vi "autonSample.vi"(0 "Auton Array":dbl[][](array[numeric]), 5 "LeftEncoder":dbl, 7 "RightEncoder":dbl, 11 "MeasuredHeading":dbl) -> (4 "Left Drive":dbl, 6 "Right Drive":dbl, 8 "Ramp ACT motor":dbl, 10 "Harvester":dbl, 13 "Shooter motor output":dbl, 14 "Turret Rotation":dbl, 15 "Convyeor":dbl)   [LabVIEW 2011]
uses:
  Robot Global Data.vi
panel:
  out "Primitive ID":i16
  out "Tzero":i64
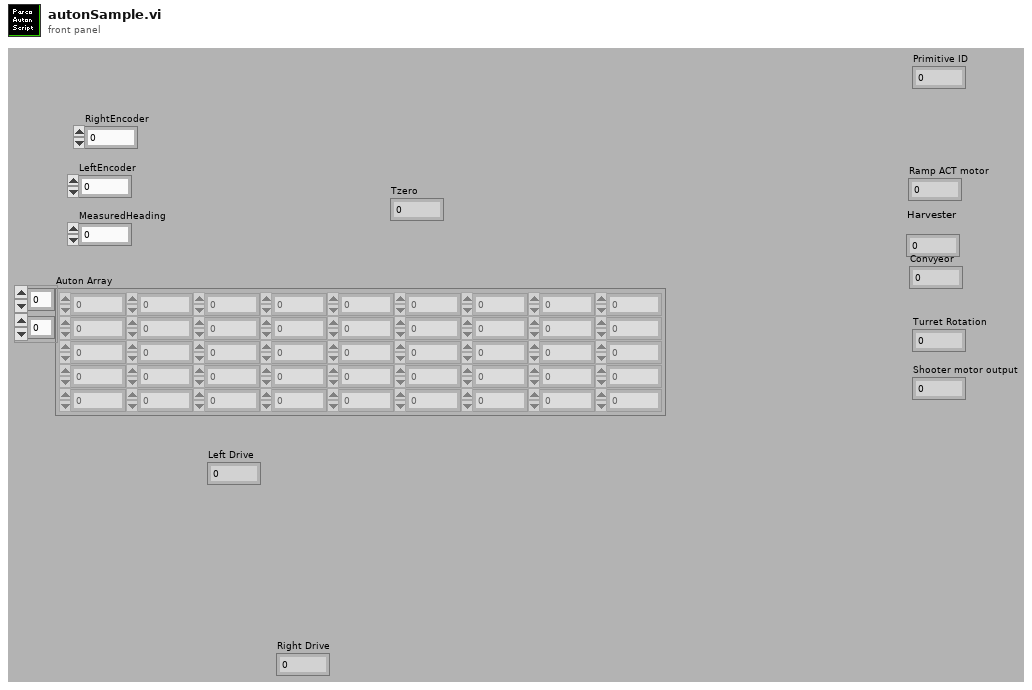
[diagram p1: front panel]
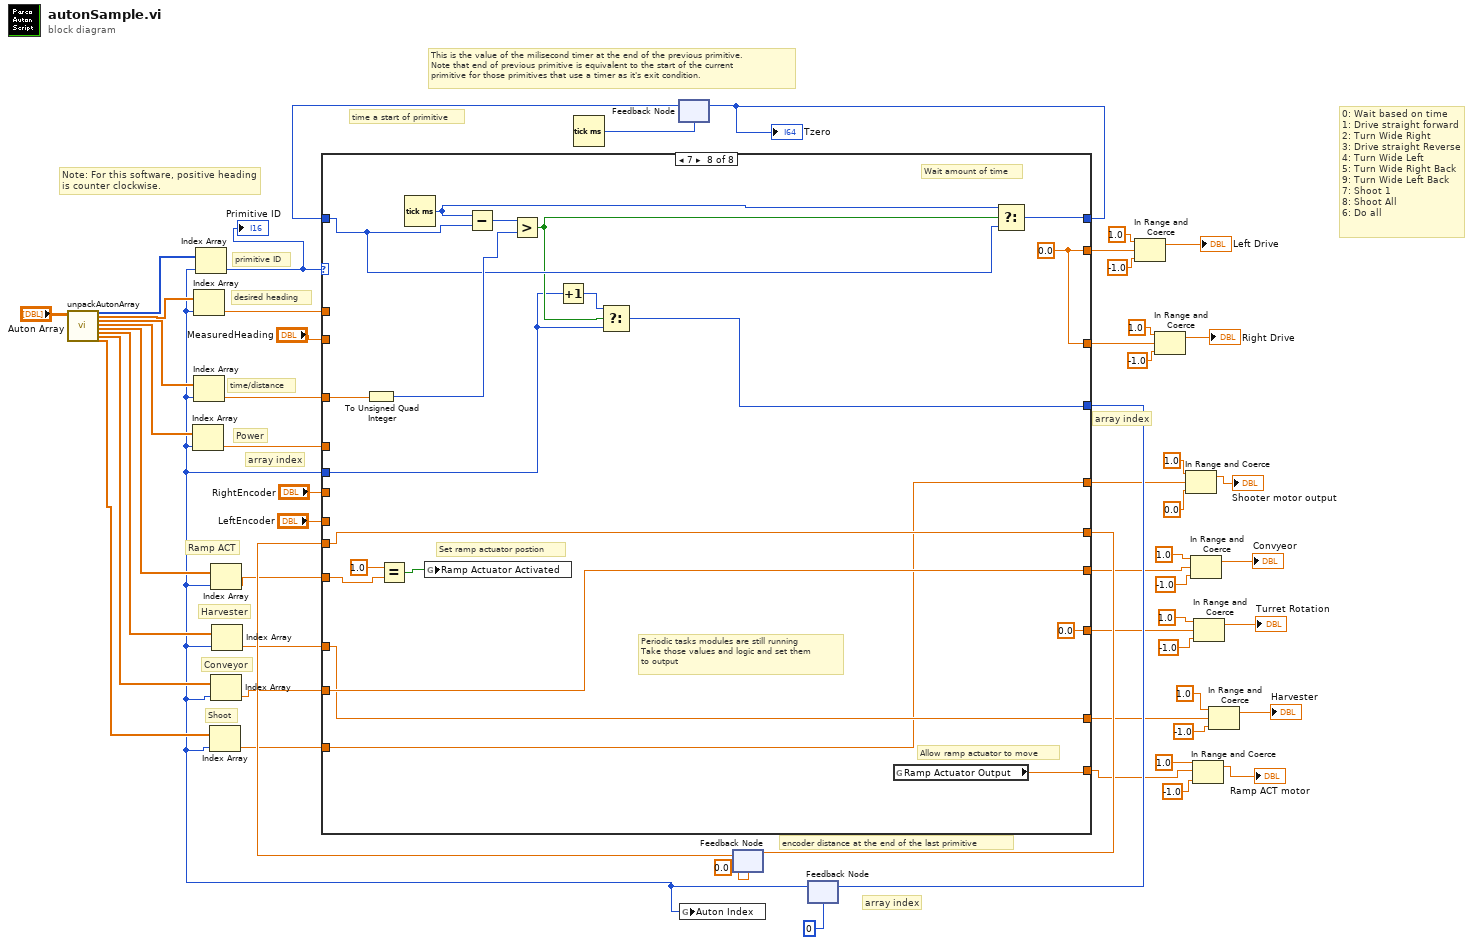
[diagram p0: block diagram]
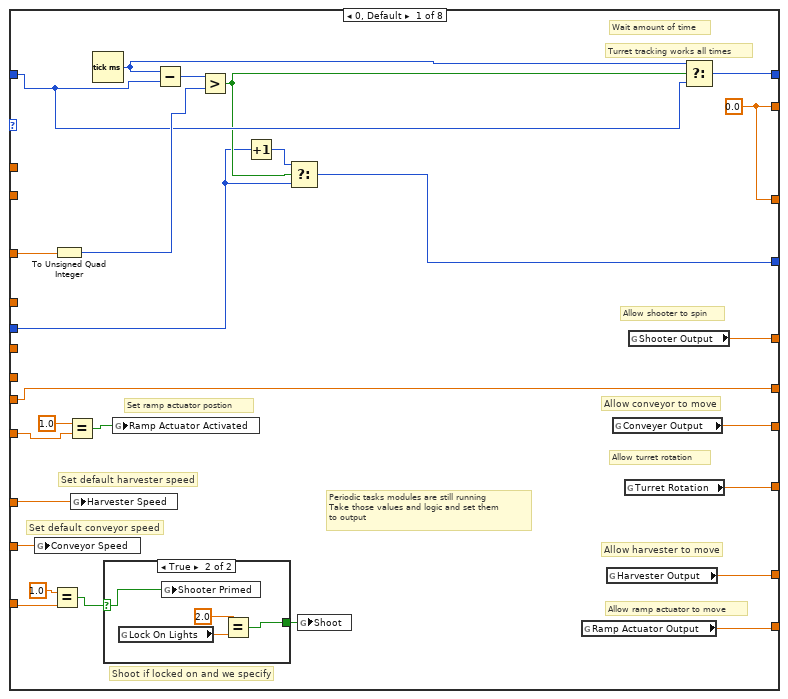
[diagram p2: hidden frame]
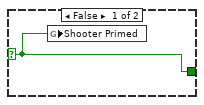
[diagram p3: hidden frame]
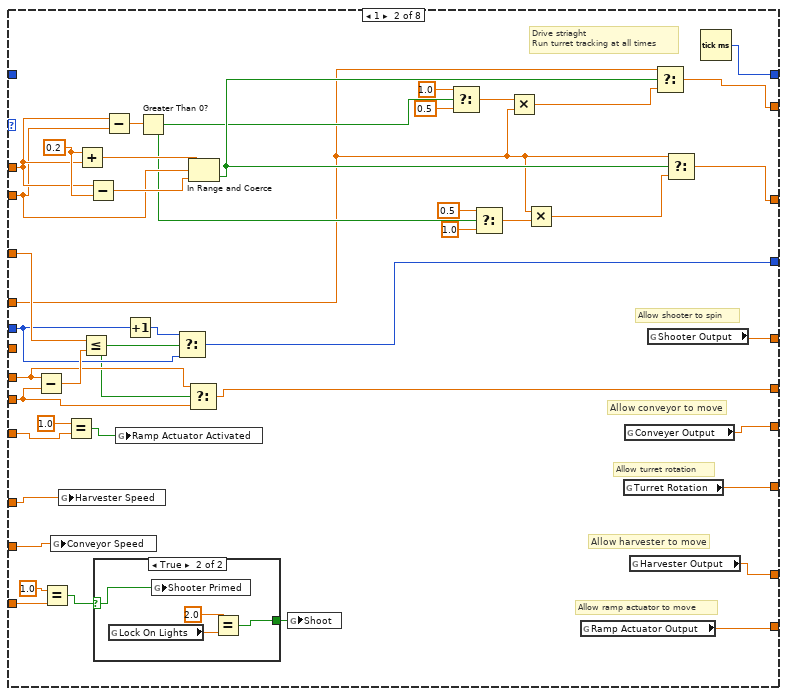
[diagram p4: hidden frame]
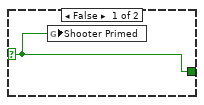
[diagram p5: hidden frame]
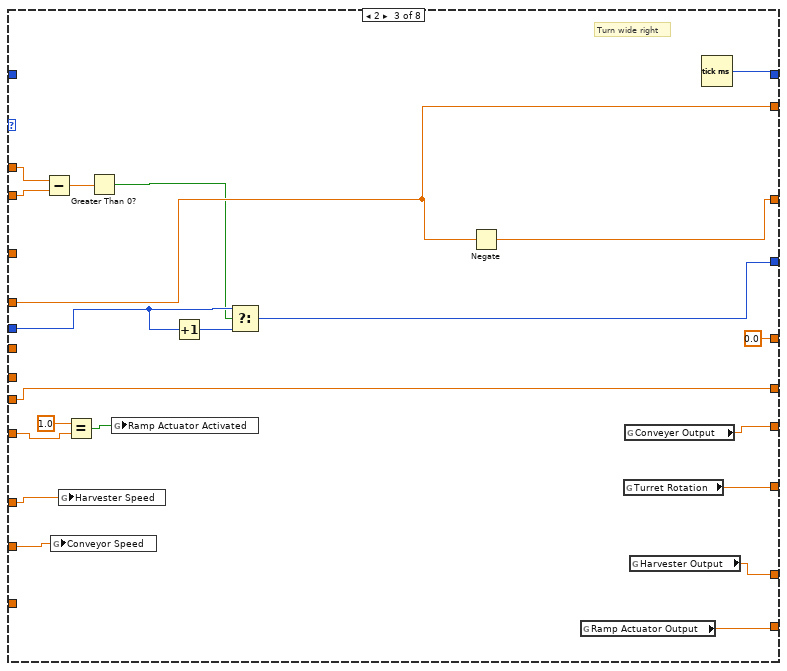
[diagram p6: hidden frame]
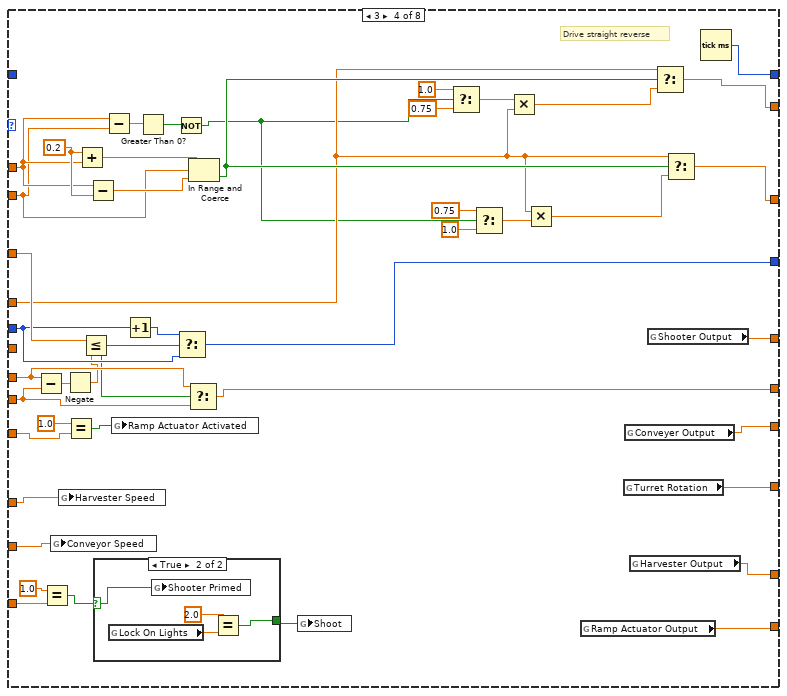
[diagram p7: hidden frame]
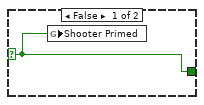
[diagram p8: hidden frame]
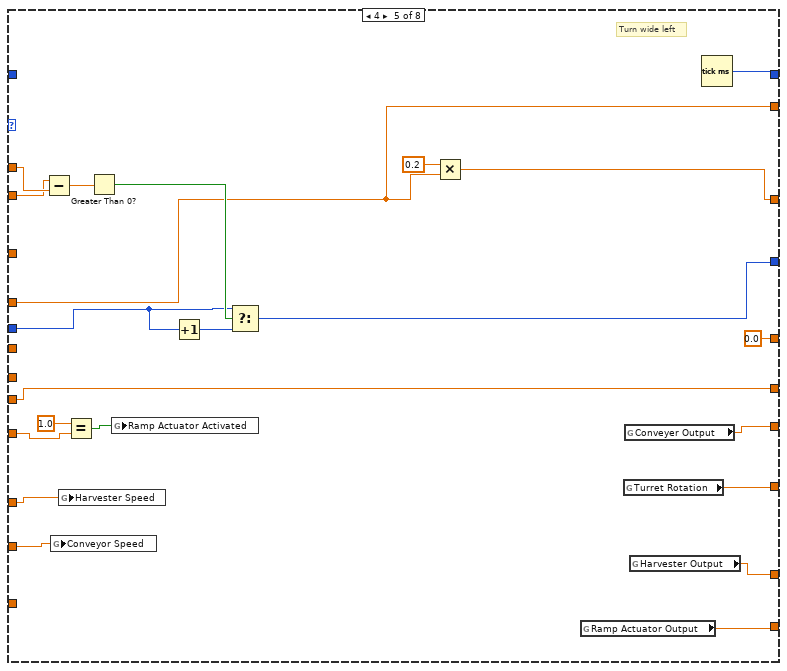
[diagram p9: hidden frame]
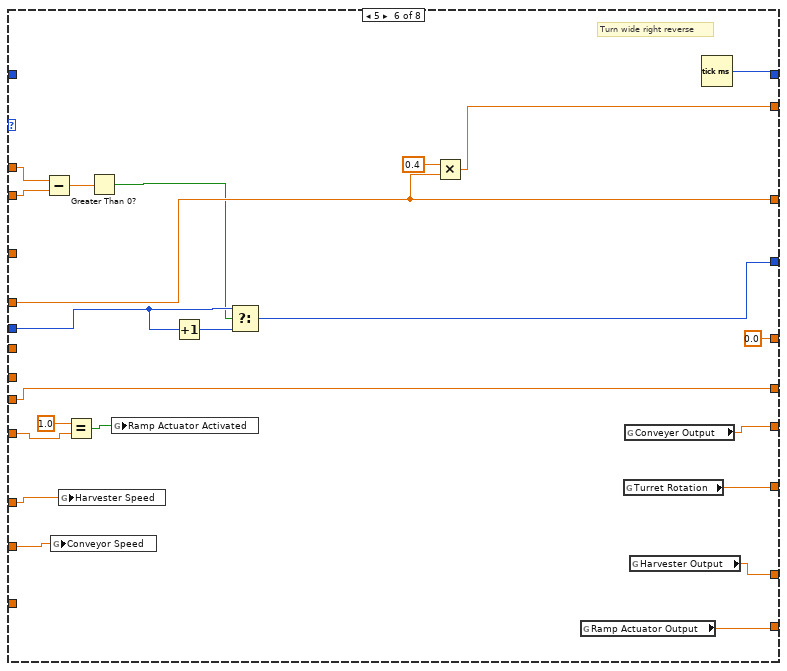
[diagram p10: hidden frame]
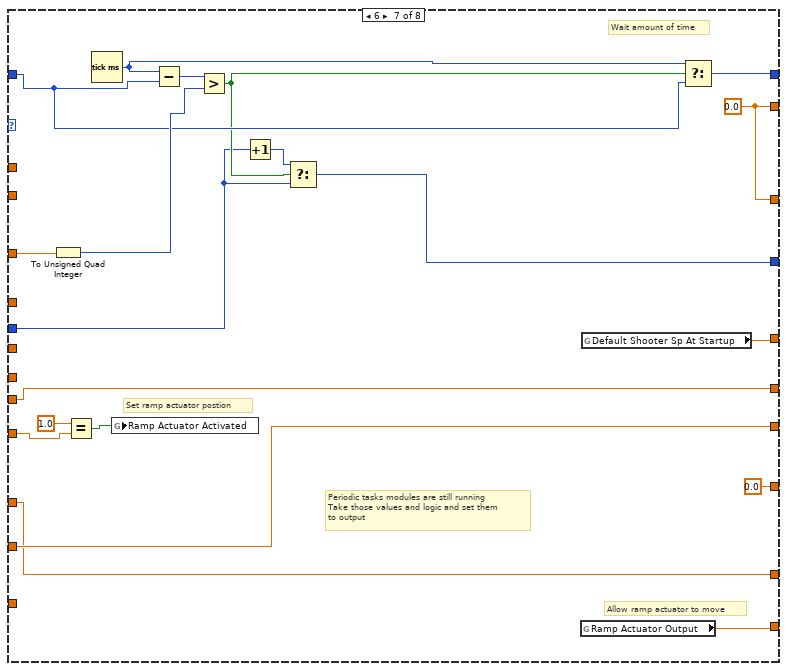
[diagram p11: hidden frame]
diagram:
  # "0: Wait based on time\n1: Drive straight forward\n2: Turn Wide Right\n3: Drive straight Reverse\n4: Turn Wide Left\n5: Turn Wide Right Back\n9: Turn Wide Left Back\n7: Shoot 1\n8: Shoot All\n6: Do all"
  # "Shoot"
  # "Conveyor"
  # "Harvester"
  # "Ramp ACT"
  # "encoder distance at the end of the last primitive"
  # "Note: For this software, positive heading\nis counter clockwise."
  # "time a start of primitive"
  # "array index"
  # "array index"
  # "This is the value of the milisecond timer at the end of the previous primitive.\nNote that end of previous primitive is equivalent to the start of the current\nprimitive for those primitives that use a timer as it's exit condition."
  # "Power"
  # "array index"
  # "desired heading"
  # "primitive ID"
  # "time/distance"
  n1 = call "unpackAutonArray.vi"("all rows"="Auton Array") -> ("Primitive"=w56:i16[], "Desired Heading"=w16:dbl[], "Time/Distance"=w15:dbl[], "Power"=w14:dbl[], "Ramp Actuator"=w13:dbl[], "Harvester"=w12:dbl[], "Conveyor"=w11:dbl[], "Shoot"=w10:dbl[])  [unwired: 1 in, 18 out]
  n2 = Tick Count (ms)() -> (millisecond timer value=w51:u32)
  n3 = feedback #1(w51) -> (w55:u32)
  n4 = feedback #2(0.0 ("EncoderDistance")) -> (w39:dbl)
  n5 = feedback #3(0) -> (w8:i32)
  n6 = Index Array(array=w14, index=w8) -> (element=w53:dbl)
  n7 = Index Array(array=w16, index=w8) -> (element=w40:dbl)
  n8 = Index Array(array=w15, index=w8) -> (element=w54:dbl)
  n9 = Index Array(array=w56, index=w8) -> (element=w22:i16)
  "Primitive ID" <- w22
  n10 = Index Array(array=w10, index=w8) -> (element=w9:dbl)
  n11 = Index Array(array=w13, index=w8) -> (element=w21:dbl)
  n12 = Index Array(array=w11, index=w8) -> (element=w6:dbl)
  n13 = Index Array(array=w12, index=w8) -> (element=w7:dbl)
  n14 = case shown="7" w22 {
    tunnel: [w75 w114 w140 w186 w213 w231 w263 w283] -> w35
    tunnel: w8 -> [w76 w116 w142 w188 w215 w233 w264 w284]
    tunnel: [w83 w92 w146 w165 w219 w240 w271 w291] -> w41
    tunnel: w55 -> [w80 _ _ _ _ _ w268 w288]
    tunnel: w54 -> [w69 w117 _ w189 _ _ w258 w278]
    tunnel: w40 -> [_ w105 w145 w177 w210 w239 _ _]
    tunnel: [w74 w91 w139 w164 w212 w235 w262 w282] -> w49
    tunnel: [w74 w90 w138 w163 w211 w237 w262 w282] -> w42
    tunnel: w53 -> [_ w94 w139 w167 w212 w237 _ _]
    tunnel: "LeftEncoder" -> [_ w111 _ w183 _ _ _ _]
    tunnel: "MeasuredHeading" -> [_ w104 w144 w176 w209 w238 _ _]
    tunnel: [w68 w113 w148 w185 w221 w242 w257 w277] -> w36
    tunnel: w39 -> [w68 w112 w148 w184 w221 w242 w257 w277]
    tunnel: [w58 w119 0.0 ("Shooter Output") w190 0.0 ("Shooter Output") 0.0 ("Shooter Output") w252 w272] -> w31
    tunnel: [w70 w129 w154 w199 w226 w248 0.0 ("Turret Rotation") 0.0 ("Turret Rotation")] -> w27
    tunnel: [w66 w123 w150 w194 w223 w244 w254 w274] -> w23
    tunnel: w21 -> [w63 w126 w153 w162 w208 w247 w256 w276]
    tunnel: [w71 w130 w155 w200 w227 w249 w259 w279] -> w20
    tunnel: w9 -> [w59 w127 _ w197 _ _ _ w272]
    tunnel: w7 -> [w64 w125 w152 w196 w225 w246 w254 w274]
    tunnel: w6 -> [w65 w124 w151 w195 w224 w245 w255 w275]
    tunnel: [w67 w122 w149 w193 w222 w243 w255 w275] -> w2
    tunnel: "RightEncoder" -> [_ _ _ _ _ _ _ _]
    frame 0, Default {
      w74 = 0.0 ("Numeric")
      # "Periodic tasks modules are still running\nTake those values and logic and set them \nto output"
      # "Set ramp actuator postion"
      # "Set default harvester speed"
      # "Set default conveyor speed"
      # "Shoot if locked on and we specify"
      # "Allow ramp actuator to move"
      # "Allow harvester to move"
      # "Turret tracking works all times"
      # "Allow turret rotation"
      # "Allow conveyor to move"
      # "Allow shooter to spin"
      # "Wait amount of time"
      n15 = global write "Robot Global Data.vi" "Conveyor Speed"(w65) -> ()
      n16 = Equal?(x=1.0, y=w59) -> (x = y?=w61:bool)
      n17 = To Unsigned Quad Integer(1:w69) -> (0:w81:u64)
      n18 = Equal?(x=1.0, y=w63) -> (x = y?=w72:bool)
      n19 = global write "Robot Global Data.vi" "Harvester Speed"(w64) -> ()
      n20 = Tick Count (ms)() -> (millisecond timer value=w79:u32)
      n21 = case shown="True" w61 {
        selector: w61 -> [w84 w88]
        tunnel: [w84 w85] -> w60
        frame False {
          n22 = global write "Robot Global Data.vi" "Shooter Primed"(w84) -> ()
        }
        frame True {
          n23 = global read "Robot Global Data.vi" "Lock On Lights"() -> (w86:dbl)
          n24 = global write "Robot Global Data.vi" "Shooter Primed"(w88) -> ()
          n25 = Equal?(x=2.0, y=w86) -> (x = y?=w85:bool)
        }
      }
      n26 = global write "Robot Global Data.vi" "Ramp Actuator Activated"(w72) -> ()
      n27 = Subtract(x=w79, y=w80) -> (x-y=w82:u32)
      n28 = Greater?(x=w82, y=w81) -> (0:w78:bool)
      n29 = Increment(x=w76) -> (x+1=w77:i32)
      n30 = Select(t=w77, s=w78, f=w76) -> (s? t:f=w75:i32)
      n31 = global write "Robot Global Data.vi" "Shoot"(w60) -> ()
      n32 = global read "Robot Global Data.vi" "Ramp Actuator Output"() -> (w71:dbl)
      n33 = global read "Robot Global Data.vi" "Harvester Output"() -> (w66:dbl)
      n34 = global read "Robot Global Data.vi" "Conveyer Output"() -> (w67:dbl)
      n35 = global read "Robot Global Data.vi" "Turret Rotation"() -> (w70:dbl)
      n36 = global read "Robot Global Data.vi" "Shooter Output"() -> (w58:dbl)
      n37 = Select(t=w79, s=w78, f=w80) -> (s? t:f=w83:u32)
    }
    frame 1 {
      w109 = 0.2 ("x")
      # "Allow ramp actuator to move"
      # "Allow harvester to move"
      # "Allow turret rotation"
      # "Allow conveyor to move"
      # "Allow shooter to spin"
      # "Drive striaght\nRun turret tracking at all times"
      n38 = Subtract(x=w111, y=w112) -> (x-y=w118:dbl)
      n39 = Equal?(x=1.0, y=w127) -> (x = y?=w121:bool)
      n40 = global write "Robot Global Data.vi" "Conveyor Speed"(w124) -> ()
      n41 = global write "Robot Global Data.vi" "Harvester Speed"(w125) -> ()
      n42 = Equal?(x=1.0, y=w126) -> (x = y?=w89:bool)
      n43 = Add(x=w109, y=w105) -> (x+y=w107:dbl)
      n44 = Less Or Equal?(x=w117, y=w118) -> (x <= y?=w110:bool)
      n45 = Subtract(x=w105, y=w109) -> (x-y=w108:dbl)
      n46 = case shown="True" w121 {
        selector: w121 -> [w132 w136]
        tunnel: [w132 w133] -> w120
        frame False {
          n47 = global write "Robot Global Data.vi" "Shooter Primed"(w132) -> ()
        }
        frame True {
          n48 = global read "Robot Global Data.vi" "Lock On Lights"() -> (w134:dbl)
          n49 = global write "Robot Global Data.vi" "Shooter Primed"(w136) -> ()
          n50 = Equal?(x=2.0, y=w134) -> (x = y?=w133:bool)
        }
      }
      n51 = Subtract(x=w105, y=w104) -> (x-y=w103:dbl)
      n52 = global write "Robot Global Data.vi" "Ramp Actuator Activated"(w89) -> ()
      n53 = Increment(x=w116) -> (x+1=w115:i32)
      n54 = Greater Than 0?(x=w103) -> (x > 0?=w102:bool)
      n55 = Select(t=w115, s=w110, f=w116) -> (s? t:f=w114:i32)
      n56 = Select(t=w111, s=w110, f=w112) -> (s? t:f=w113:dbl)
      n57 = In Range and Coerce(upper limit=w107, x=w104, lower limit=w108) -> (In Range?=w106:bool)  [unwired: 1 out]
      n58 = global write "Robot Global Data.vi" "Shoot"(w120) -> ()
      n59 = Select(t=1.0, s=w102, f=0.5) -> (s? t:f=w95:dbl)
      n60 = Select(t=0.5, s=w102, f=1.0) -> (s? t:f=w97:dbl)
      n61 = Multiply(x=w95, y=w94) -> (x*y=w93:dbl)
      n62 = Multiply(x=w94, y=w97) -> (x*y=w96:dbl)
      n63 = global read "Robot Global Data.vi" "Ramp Actuator Output"() -> (w130:dbl)
      n64 = global read "Robot Global Data.vi" "Turret Rotation"() -> (w129:dbl)
      n65 = global read "Robot Global Data.vi" "Conveyer Output"() -> (w122:dbl)
      n66 = global read "Robot Global Data.vi" "Harvester Output"() -> (w123:dbl)
      n67 = global read "Robot Global Data.vi" "Shooter Output"() -> (w119:dbl)
      n68 = Select(t=w94, s=w106, f=w93) -> (s? t:f=w91:dbl)
      n69 = Select(t=w94, s=w106, f=w96) -> (s? t:f=w90:dbl)
      n70 = Tick Count (ms)() -> (millisecond timer value=w92:u32)
    }
    frame 2 {
      # "Turn wide right"
      n71 = Subtract(x=w145, y=w144) -> (x-y=w143:dbl)
      n72 = global write "Robot Global Data.vi" "Conveyor Speed"(w151) -> ()
      n73 = global write "Robot Global Data.vi" "Harvester Speed"(w152) -> ()
      n74 = Equal?(x=1.0, y=w153) -> (x = y?=w156:bool)
      n75 = Greater Than 0?(x=w143) -> (x > 0?=w137:bool)
      n76 = global write "Robot Global Data.vi" "Ramp Actuator Activated"(w156) -> ()
      n77 = Increment(x=w142) -> (x+1=w141:i32)
      n78 = Select(t=w142, s=w137, f=w141) -> (s? t:f=w140:i32)
      n79 = Negate(x=w139) -> (-x=w138:dbl)
      n80 = global read "Robot Global Data.vi" "Ramp Actuator Output"() -> (w155:dbl)
      n81 = global read "Robot Global Data.vi" "Turret Rotation"() -> (w154:dbl)
      n82 = global read "Robot Global Data.vi" "Conveyer Output"() -> (w149:dbl)
      n83 = global read "Robot Global Data.vi" "Harvester Output"() -> (w150:dbl)
      n84 = Tick Count (ms)() -> (millisecond timer value=w146:u32)
    }
    frame 3 {
      w181 = 0.2 ("x")
      # "Drive straight reverse"
      n85 = Subtract(x=w183, y=w184) -> (x-y=w161:dbl)
      n86 = Equal?(x=1.0, y=w197) -> (x = y?=w192:bool)
      n87 = global write "Robot Global Data.vi" "Conveyor Speed"(w195) -> ()
      n88 = global write "Robot Global Data.vi" "Harvester Speed"(w196) -> ()
      n89 = Negate(x=w161) -> (-x=w160:dbl)
      n90 = Equal?(x=1.0, y=w162) -> (x = y?=w201:bool)
      n91 = Add(x=w181, y=w177) -> (x+y=w179:dbl)
      n92 = Less Or Equal?(x=w189, y=w160) -> (x <= y?=w182:bool)
      n93 = Subtract(x=w177, y=w181) -> (x-y=w180:dbl)
      n94 = case shown="True" w192 {
        selector: w192 -> [w203 w207]
        tunnel: [w203 w204] -> w191
        frame False {
          n95 = global write "Robot Global Data.vi" "Shooter Primed"(w203) -> ()
        }
        frame True {
          n96 = global read "Robot Global Data.vi" "Lock On Lights"() -> (w205:dbl)
          n97 = global write "Robot Global Data.vi" "Shooter Primed"(w207) -> ()
          n98 = Equal?(x=2.0, y=w205) -> (x = y?=w204:bool)
        }
      }
      n99 = Subtract(x=w177, y=w176) -> (x-y=w175:dbl)
      n100 = global write "Robot Global Data.vi" "Ramp Actuator Activated"(w201) -> ()
      n101 = Increment(x=w188) -> (x+1=w187:i32)
      n102 = Greater Than 0?(x=w175) -> (x > 0?=w159:bool)
      n103 = Not(x=w159) -> (.not. x?=w158:bool)
      n104 = Select(t=w187, s=w182, f=w188) -> (s? t:f=w186:i32)
      n105 = Select(t=w183, s=w182, f=w184) -> (s? t:f=w185:dbl)
      n106 = In Range and Coerce(upper limit=w179, x=w176, lower limit=w180) -> (In Range?=w178:bool)  [unwired: 1 out]
      n107 = global write "Robot Global Data.vi" "Shoot"(w191) -> ()
      n108 = Select(t=1.0, s=w158, f=0.75) -> (s? t:f=w168:dbl)
      n109 = Select(t=0.75, s=w158, f=1.0) -> (s? t:f=w170:dbl)
      n110 = Multiply(x=w168, y=w167) -> (x*y=w166:dbl)
      n111 = Multiply(x=w167, y=w170) -> (x*y=w169:dbl)
      n112 = global read "Robot Global Data.vi" "Ramp Actuator Output"() -> (w200:dbl)
      n113 = global read "Robot Global Data.vi" "Turret Rotation"() -> (w199:dbl)
      n114 = global read "Robot Global Data.vi" "Conveyer Output"() -> (w193:dbl)
      n115 = global read "Robot Global Data.vi" "Harvester Output"() -> (w194:dbl)
      n116 = global read "Robot Global Data.vi" "Shooter Output"() -> (w190:dbl)
      n117 = Select(t=w167, s=w178, f=w166) -> (s? t:f=w164:dbl)
      n118 = Select(t=w167, s=w178, f=w169) -> (s? t:f=w163:dbl)
      n119 = Tick Count (ms)() -> (millisecond timer value=w165:u32)
    }
    frame 4 {
      # "Turn wide left"
      n120 = Subtract(x=w209, y=w210) -> (x-y=w217:dbl)
      n121 = global write "Robot Global Data.vi" "Conveyor Speed"(w224) -> ()
      n122 = global write "Robot Global Data.vi" "Harvester Speed"(w225) -> ()
      n123 = Equal?(x=1.0, y=w208) -> (x = y?=w228:bool)
      n124 = Greater Than 0?(x=w217) -> (x > 0?=w216:bool)
      n125 = global write "Robot Global Data.vi" "Ramp Actuator Activated"(w228) -> ()
      n126 = Increment(x=w215) -> (x+1=w214:i32)
      n127 = Select(t=w215, s=w216, f=w214) -> (s? t:f=w213:i32)
      n128 = Multiply(x=0.2, y=w212) -> (x*y=w211:dbl)
      n129 = global read "Robot Global Data.vi" "Ramp Actuator Output"() -> (w227:dbl)
      n130 = global read "Robot Global Data.vi" "Turret Rotation"() -> (w226:dbl)
      n131 = global read "Robot Global Data.vi" "Conveyer Output"() -> (w222:dbl)
      n132 = global read "Robot Global Data.vi" "Harvester Output"() -> (w223:dbl)
      n133 = Tick Count (ms)() -> (millisecond timer value=w219:u32)
    }
    frame 5 {
      # "Turn wide right reverse"
      n134 = Subtract(x=w239, y=w238) -> (x-y=w234:dbl)
      n135 = global write "Robot Global Data.vi" "Conveyor Speed"(w245) -> ()
      n136 = global write "Robot Global Data.vi" "Harvester Speed"(w246) -> ()
      n137 = Equal?(x=1.0, y=w247) -> (x = y?=w250:bool)
      n138 = Greater Than 0?(x=w234) -> (x > 0?=w230:bool)
      n139 = global write "Robot Global Data.vi" "Ramp Actuator Activated"(w250) -> ()
      n140 = Increment(x=w233) -> (x+1=w232:i32)
      n141 = Select(t=w233, s=w230, f=w232) -> (s? t:f=w231:i32)
      n142 = Multiply(x=0.4, y=w237) -> (x*y=w235:dbl)
      n143 = global read "Robot Global Data.vi" "Ramp Actuator Output"() -> (w249:dbl)
      n144 = global read "Robot Global Data.vi" "Turret Rotation"() -> (w248:dbl)
      n145 = global read "Robot Global Data.vi" "Conveyer Output"() -> (w243:dbl)
      n146 = global read "Robot Global Data.vi" "Harvester Output"() -> (w244:dbl)
      n147 = Tick Count (ms)() -> (millisecond timer value=w240:u32)
    }
    frame 6 {
      w262 = 0.0 ("Numeric")
      # "Periodic tasks modules are still running\nTake those values and logic and set them \nto output"
      # "Set ramp actuator postion"
      # "Allow ramp actuator to move"
      # "Wait amount of time"
      n148 = To Unsigned Quad Integer(1:w258) -> (0:w269:u64)
      n149 = Equal?(x=1.0, y=w256) -> (x = y?=w260:bool)
      n150 = Tick Count (ms)() -> (millisecond timer value=w267:u32)
      n151 = global write "Robot Global Data.vi" "Ramp Actuator Activated"(w260) -> ()
      n152 = Subtract(x=w267, y=w268) -> (x-y=w270:u32)
      n153 = Greater?(x=w270, y=w269) -> (0:w266:bool)
      n154 = Increment(x=w264) -> (x+1=w265:i32)
      n155 = Select(t=w265, s=w266, f=w264) -> (s? t:f=w263:i32)
      n156 = global read "Robot Global Data.vi" "Ramp Actuator Output"() -> (w259:dbl)
      n157 = global read "Robot Global Data.vi" "Default Shooter Sp At Startup"() -> (w252:dbl)
      n158 = Select(t=w267, s=w266, f=w268) -> (s? t:f=w271:u32)
    }
    frame 7 {
      w282 = 0.0 ("Numeric")
      # "Periodic tasks modules are still running\nTake those values and logic and set them \nto output"
      # "Set ramp actuator postion"
      # "Allow ramp actuator to move"
      # "Wait amount of time"
      n159 = To Unsigned Quad Integer(1:w278) -> (0:w289:u64)
      n160 = Equal?(x=1.0, y=w276) -> (x = y?=w280:bool)
      n161 = Tick Count (ms)() -> (millisecond timer value=w287:u32)
      n162 = global write "Robot Global Data.vi" "Ramp Actuator Activated"(w280) -> ()
      n163 = Subtract(x=w287, y=w288) -> (x-y=w290:u32)
      n164 = Greater?(x=w290, y=w289) -> (0:w286:bool)
      n165 = Increment(x=w284) -> (x+1=w285:i32)
      n166 = Select(t=w285, s=w286, f=w284) -> (s? t:f=w283:i32)
      n167 = global read "Robot Global Data.vi" "Ramp Actuator Output"() -> (w279:dbl)
      n168 = Select(t=w287, s=w286, f=w288) -> (s? t:f=w291:u32)
    }
  }
  "Tzero" <- w41
  n169 = feedback-in #1(w41) -> ()
  n170 = global write "Robot Global Data.vi" "Auton Index"(w8) -> ()
  n171 = feedback-in #2(w36) -> ()
  n172 = feedback-in #3(w35) -> ()
  n173 = In Range and Coerce(upper limit=1.0, x=w49, lower limit=-1.0) -> (coerced(x)=→"Left Drive":dbl)  [unwired: 1 out]
  n174 = In Range and Coerce(upper limit=1.0, x=w42, lower limit=-1.0) -> (coerced(x)=→"Right Drive":dbl)  [unwired: 1 out]
  n175 = In Range and Coerce(upper limit=1.0, x=w31, lower limit=0.0) -> (coerced(x)=→"Shooter motor output":dbl)  [unwired: 1 out]
  n176 = In Range and Coerce(upper limit=1.0, x=w2, lower limit=-1.0) -> (coerced(x)=→"Convyeor":dbl)  [unwired: 1 out]
  n177 = In Range and Coerce(upper limit=1.0, x=w20, lower limit=-1.0) -> (coerced(x)=→"Ramp ACT motor":dbl)  [unwired: 1 out]
  n178 = In Range and Coerce(upper limit=1.0, x=w27, lower limit=-1.0) -> (coerced(x)=→"Turret Rotation":dbl)  [unwired: 1 out]
  n179 = In Range and Coerce(upper limit=1.0, x=w23, lower limit=-1.0) -> (coerced(x)=→"Harvester":dbl)  [unwired: 1 out]
